vi "GetServerRef.vi"(8 "error in":errorcluster, 10 "Force Destroy (F)":bool, 11 "Destroy (F)":bool) -> (0 "error out":errorcluster, 2 "Server":refnum<class "Server.lvclass">, 3 "Created":bool)   [LabVIEW 2013]
uses:
  source/Server/Server class/Server.lvclass
  source/Server/Server class/Server.lvclass/Server.ctl
  source/MQTT_Base/MQTT_Base.lvclass
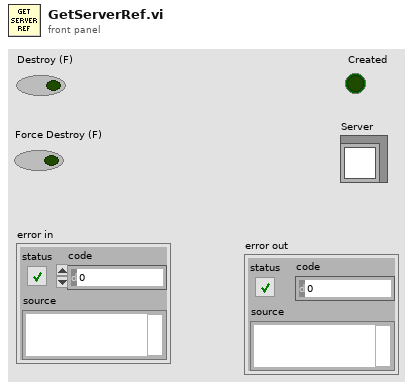
[diagram p1: front panel]
types:
  T1 = typedef "MQTT Server.lvlib/Server.lvclass/Public Events -- cluster.ctl" = cluster{"NbConnections":refnum<user-event>}
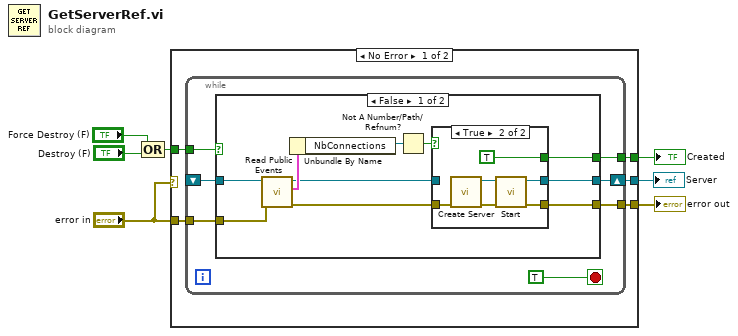
[diagram p0: block diagram]
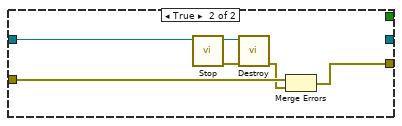
[diagram p3: hidden frame]
diagram:
  n1 = Compound Arithmetic op=OR("Force Destroy (F)", "Destroy (F)") -> (w3:bool)
  n2 = case shown="No Error" "error in" {
    tunnel: [w12 _] -> w7
    tunnel: [w11 _] -> w6
    tunnel: [w10 w44] -> w5
    tunnel: "error in" -> [w9 w44]
    tunnel: w3 -> [w8 _]
    frame No Error {
      n3 = while {
        shift-right: [w18] -> w12
        shift-left: _ -> [w15]
        tunnel: [w17] -> w11
        tunnel: w8 -> [w16]
        tunnel: [w14] -> w10
        tunnel: w9 -> [w13]
        stop <- TRUE stop-if-true
        n4 = case shown="False" w16 {
          tunnel: [w29 _] -> w18
          tunnel: [w28 w38] -> w14
          tunnel: [w27 _] -> w17
          tunnel: w15 -> [w26 w41]
          tunnel: w13 -> [w20 w40]
          frame False {
            n5 = call "Read Public Events.vi"("error in (no error)"=w20, "Server in"=w26) -> ("error out"=w21:errorcluster, "Public Events"=w25:T1, "Server out"=w22:refnum<class "Server.lvclass">)  [unwired: 7 in]
            n6 = Unbundle By Name(w25) -> ("NbConnections"=w24:refnum<user-event>)
            n7 = Not A Number/Path/Refnum?(number/path/refnum=w24) -> (NaN/Path/Refnum?=w23:bool)
            n8 = case shown="True" w23 {
              tunnel: [w31 w35] -> w29
              tunnel: [w30 w34] -> w28
              tunnel: [_ TRUE] -> w27
              tunnel: w22 -> [w31 _]
              tunnel: w21 -> [w30 w32]
              frame False {
              }
              frame True {
                n9 = call "Create Server.vi"("error in (no error)"=w32) -> ("error out"=w36:errorcluster, "Server"=w37:refnum<class "Server.lvclass">)  [unwired: 9 in]
                n10 = call "Start.vi"("error in (no error)"=w36, "MQTT_Base in"=w37) -> ("error out"=w34:errorcluster, "MQTT_Base out"=w35:refnum<class "Server.lvclass">)  [unwired: 7 in, 1 out]
              }
            }
          }
          frame True {
            n11 = call "Stop.vi"("MQTT_Base in"=w41) -> ("error out"=w42:errorcluster, "MQTT_Base out"=w43:refnum<class "Server.lvclass">)  [unwired: 8 in, 1 out]
            n12 = call-dynamic "Destroy.vi"("error in (no error)"=w42, "Server in"=w43) -> ("error out"=w39:errorcluster)  [unwired: 8 in, 1 out]
            n13 = Merge Errors(w40, w39) -> (w38:errorcluster)
          }
        }
      }
    }
    frame Error {
    }
  }
  "Server" <- w7
  "Created" <- w6
  "error out" <- w5
